vi "FGV Ventile manuell steuern.vi"(0 "Ventile schalten":u32, 11 "error in (no error)":errorcluster caption="Fehler (Eingang, kein Fehler)", 13 "Aktion":T1) -> (4 "Ventile schalten":u32, 15 "error out":errorcluster caption="Fehler (Ausgang)")   [LabVIEW 2020, in "PNS.lvlib"]
uses:
  PNS.lvlib
  Aktion FGV Ventile manuell steuern.ctl
panel:
  # "Version HP(normal)\nZustand+Anweisungscode               Ventilansteuerungs zahl\nSpülen Filter                                     1 und 3 wechseln\nCalGas                                             4\nMessen 1                                         16      \nCalGasOverflow                                6\nSpülen Leitung 1                               17\nLüften                                               2\nMessen 2                                         32              \nSpülen 2                                           33            \nMessen 3                                         64              \nSpülen 3                                           65           \nMessen 4                                         128             \nSpülen 4                                           129          \nMessen 5                                         256              \nSpülen 5                                           257           \nMessen 6                                         512             \nSpülen 6                                           513"
  # "Version LP\nZustand+Anweisungscode               Ventilansteuerungs zahl\nSpülen Filter                                      1 und 3 wechseln\nCalGas                                             1025\nMessen 1                       VFS2-6        1040      \nCalGasOverflow                                1030 \nSpülen Leitung 1                               17\nLüften                                              2\nMessen 2                                         1056              \nSpülen 2                                           33            \nMessen 3                                         1088              \nSpülen 3                                           65           \nMessen 4                                         1152             \nSpülen 4                                           129          \nMessen 5                                         1280              \nSpülen 5                                           257           \nMessen 6                                         1536             \nSpülen 6                                           513"
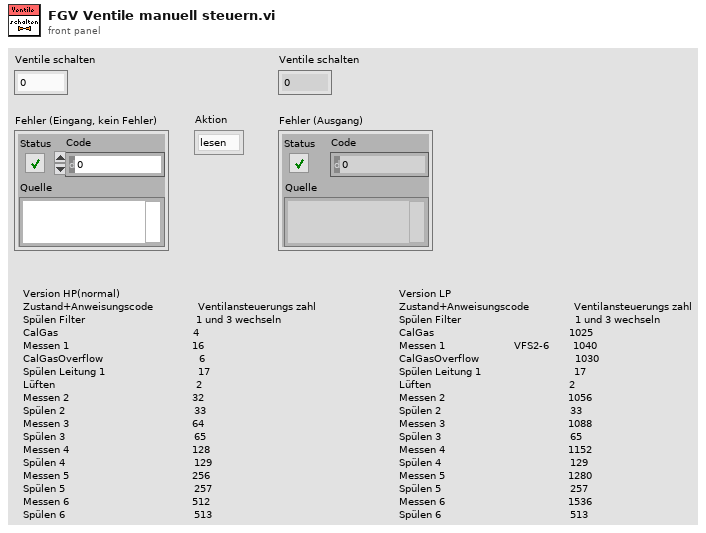
[diagram p1: front panel]
types:
  T1 = typedef "PNS.lvlib/Aktion FGV Ventile manuell steuern.ctl" = enum16{"lesen", "Ventile schalten"}
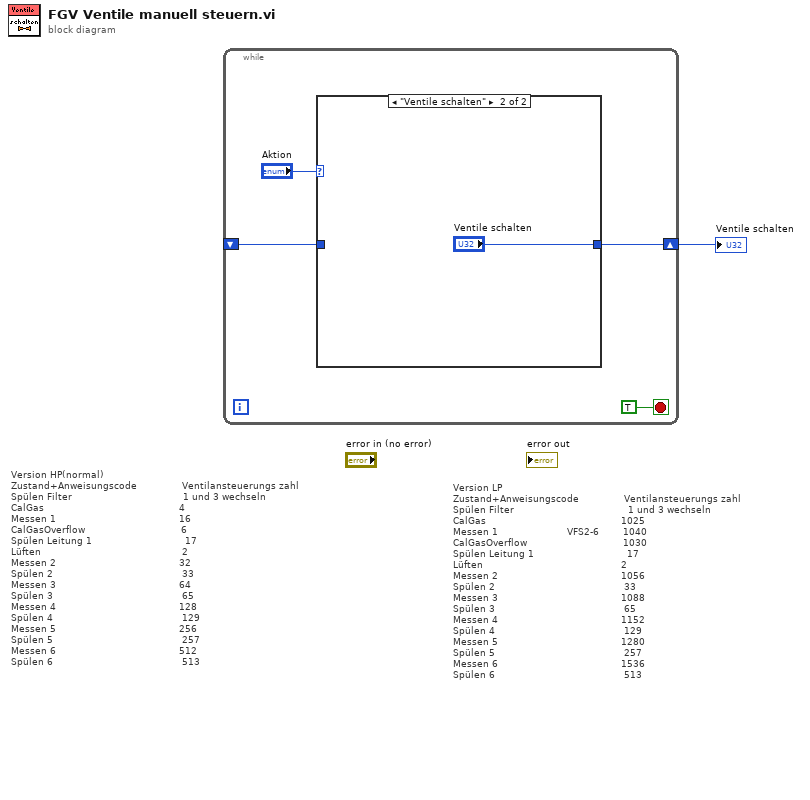
[diagram p0: block diagram]
diagram:
  # "Version LP\nZustand+Anweisungscode               Ventilansteuerungs zahl\nSpülen Filter                                      1 und 3 wechseln\nCalGas                                             1025\nMessen 1                       VFS2-6        1040      \nCalGasOverflow                                1030 \nSpülen Leitung 1                               17\nLüften                                              2\nMessen 2                                         1056              \nSpülen 2                                           33            \nMessen 3                                         1088              \nSpülen 3                                           65           \nMessen 4                                         1152             \nSpülen 4                                           129          \nMessen 5                                         1280              \nSpülen 5                                           257           \nMessen 6                                         1536             \nSpülen 6                                           513"
  # "Version HP(normal)\nZustand+Anweisungscode               Ventilansteuerungs zahl\nSpülen Filter                                     1 und 3 wechseln\nCalGas                                             4\nMessen 1                                         16      \nCalGasOverflow                                6\nSpülen Leitung 1                               17\nLüften                                               2\nMessen 2                                         32              \nSpülen 2                                           33            \nMessen 3                                         64              \nSpülen 3                                           65           \nMessen 4                                         128             \nSpülen 4                                           129          \nMessen 5                                         256              \nSpülen 5                                           257           \nMessen 6                                         512             \nSpülen 6                                           513"
  n1 = while {
    shift-right: [w3] -> w1
    shift-left: _ -> [w2]
    stop <- TRUE stop-if-true
    n2 = case shown="\"Ventile schalten\"" "Aktion" {
      tunnel: [w6 "Ventile schalten"] -> w3
      tunnel: w2 -> [w6 _]
      frame "lesen", Default {
      }
      frame "Ventile schalten" {
      }
    }
  }
  "Ventile schalten" <- w1
